vi "Purge Event Data.vi"(8 "error in":errorcluster, 11 "TDMS in":refnum<class "TDMS.lvclass">) -> (0 "error out":errorcluster, 2 "file path out":path, 3 "TDMS out":refnum<class "TDMS.lvclass">)   [LabVIEW 2019, in "TDMS.lvlib" / "TDMS.lvclass"]
uses:
  TDMS.lvclass
  TDMS.lvclass/TDMS.ctl
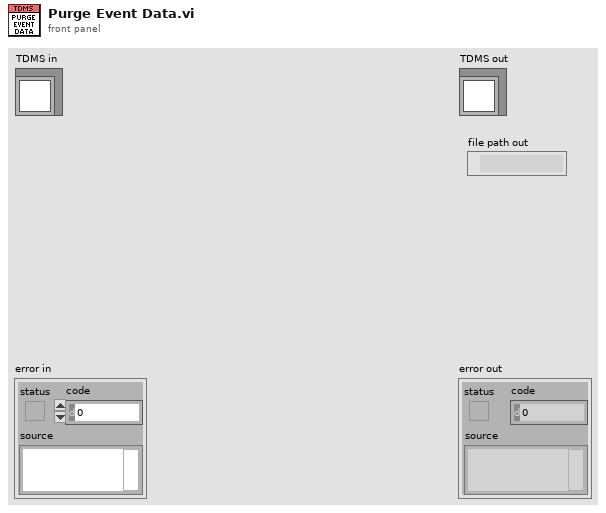
[diagram p1: front panel]
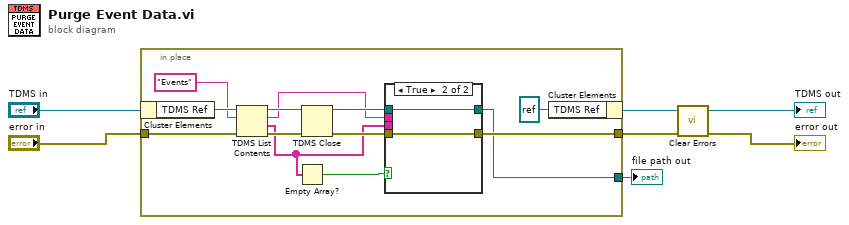
[diagram p0: block diagram]
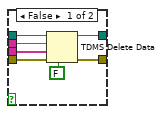
[diagram p2: hidden frame]
diagram:
  n1 = in-place {
    in-place-border: "error in" -> [w17]
    in-place-border: [w12] -> w3
    in-place-border: [w9] -> w2
    n2 = in-place-cluster #1("TDMS in") -> ("TDMS Ref"=w19:refnum<k34>)
    n3 = TDMS List Contents(4:w17, 6:"Events", 7:w19) -> (0:w15:errorcluster, 1:w8:string[], 2:w11:string, 3:w16:refnum<k34>)
    n4 = Empty Array?(array=w8) -> (empty?=w7:bool)
    n5 = TDMS Close(8:w15, 11:w16) -> (0:w13:errorcluster, 3:w14:path)
    n6 = case shown="True" w7 {
      tunnel: w14 -> [w26 w27]
      tunnel: w13 -> [w25 w28]
      tunnel: [w24 w28] -> w12
      tunnel: w11 -> [w22 _]
      tunnel: [w21 w27] -> w9
      tunnel: w8 -> [w20 _]
      frame False {
        n7 = TDMS Delete Data(6:FALSE ("keep empty group/channel? (T)"), 8:w25, 9:w20, 10:w22, 11:w26) -> (0:w24:errorcluster, 3:w21:path)  [unwired: 2 in]
      }
      frame True {
      }
    }
    n8 = in-place-cluster #1("TDMS Ref"=refnum<k34> refnum) -> (→"TDMS out":refnum<class "TDMS.lvclass">)
  }
  "file path out" <- w2
  n9 = call <vilib>:"Clear Errors.vi"("error in (no error)"=w3) -> ("error out"=→"error out":errorcluster)  [unwired: 5 in, 1 out]
